vi "destoryEvents.vi"(8 "error in (no error)":errorcluster, 11 "ScriptEdEvents in":refnum<class "ScriptEdEvents.lvclass">) -> (0 "error out":errorcluster, 3 "ScriptEdEvents out":refnum<class "ScriptEdEvents.lvclass">)   [LabVIEW 2009, in "Views.lvlib" / "ScriptEditor.lvlib" / "ScriptEdEvents.lvclass"]
uses:
  ScriptEdEvents.lvclass
  ScriptEdEvents.lvclass/ScriptEdEvents.ctl
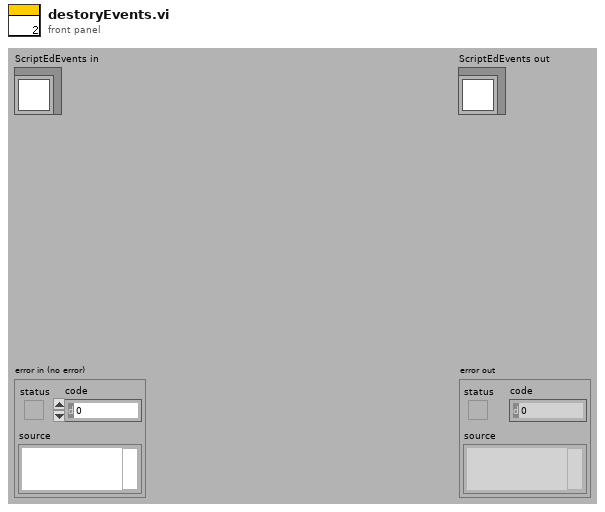
[diagram p1: front panel]
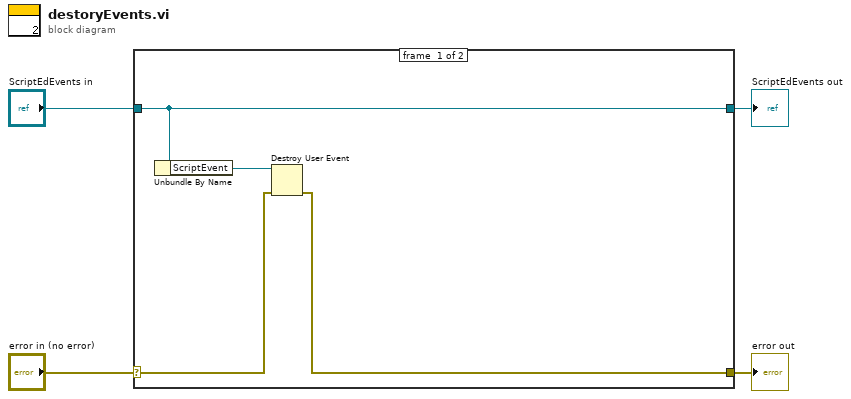
[diagram p0: block diagram]
diagram:
  n1 = case shown="No Error" "error in (no error)" {
    selector: "error in (no error)" -> [w6 w10]
    tunnel: [w5 w10] -> w3
    tunnel: [w8 w9] -> w1
    tunnel: "ScriptEdEvents in" -> [w8 w9]
    frame #0 {
      n2 = Unbundle By Name(w8) -> ("ScriptEvent"=w7:refnum<user-event>)
      n3 = Destroy User Event(user event=w7, error in=w6) -> (error out=w5:errorcluster)
    }
    frame #1 {
    }
  }
  "error out" <- w3
  "ScriptEdEvents out" <- w1
